vi "test_Bitfile Reload_Group Scalar to Group Static Scalar Data Type Change.vi"(8 "error in (no error)":errorcluster, 11 "TestCase in":refnum<class "FPGA Addon Bitfile Reload Unit Tests.lvclass">) -> (0 "error out":errorcluster, 3 "TestCase out":refnum<class "FPGA Addon Bitfile Reload Unit Tests.lvclass">)   [LabVIEW 2020, in "FPGA Addon Bitfile Reload Unit Tests.lvclass"]
uses:
  FPGA Addon Bitfile Reload Unit Tests.lvclass
  APIs/Scripting API/TypeDefs/Output Scalar Data.ctl
  Addon/Addon Shared/Types/FPGA Addon Data Type.ctl
  Addon/Addon Shared/SubVIs/Constants.vi
  APIs/Scripting API/Public/Bitfile Resources/Import Bitfile Scalars (Instances)/Import Scalars - all.vi
  <vilib>/addons/_JKI Toolkits/VI Tester/TestCase.llb/TestCase.lvclass
  FPGA Addon Test Class/FPGA Addon Test Class.lvclass
  APIs/Scripting API/Scripting API.lvlib
  Addon/Addon System Explorer/FPGA Addon System Explorer.lvlib
  Addon/Addon Shared/FPGA Addon Shared.lvlib
  C:/Program Files (x86)/National Instruments/LabVIEW 2020/vi.lib/addons/_JKI Toolkits/VI Tester/TestCase.llb/TestCase.lvclass
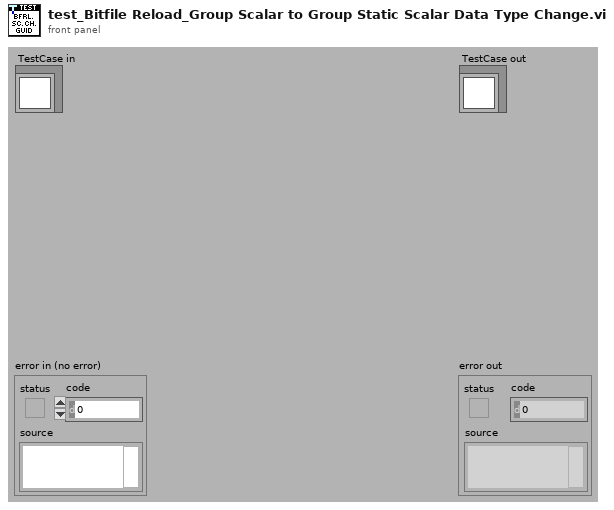
[diagram p1: front panel]
types:
  T1 = typedef "Scripting API.lvlib/Output Scalar Data.ctl" = cluster{"Bitfile Name":string, "SysDef Channel Name":string, "Imported":bool, "Data Type":T2}
  T2 = typedef "FPGA Addon Shared.lvlib/FPGA Addon Data Type.ctl" = enum8{"<Null>", "I8", "I16", "I32", "I64", "U8", "U16", "U32", "U64", "SGL", "Boolean", "Analog PWM In Settings", "Analog PWM In", "Digital PWM In Settings", "Digital PWM In", "Digital PWM Out", "Sine Out", "FXP", "FXP+/-24.5", "FXP+/-16.5", "FXP+/-32.8", "FXP+/-64.32", "FXP+/-16.7", "FXP+/-20.5", "FXP+/-27.5", "FXP+/-32.16", "FXP+16.3", "FXP+18.3", "Digital Static In", "Digital Static Out", "Digital Static In Settings", "Digital WSS Out", "Quad Encoder Settings", "Quad Encoder In", "Group"}
  T3 = typedef "Custom Device API.lvlib/Custom Device Item Ref.ctl" = u64
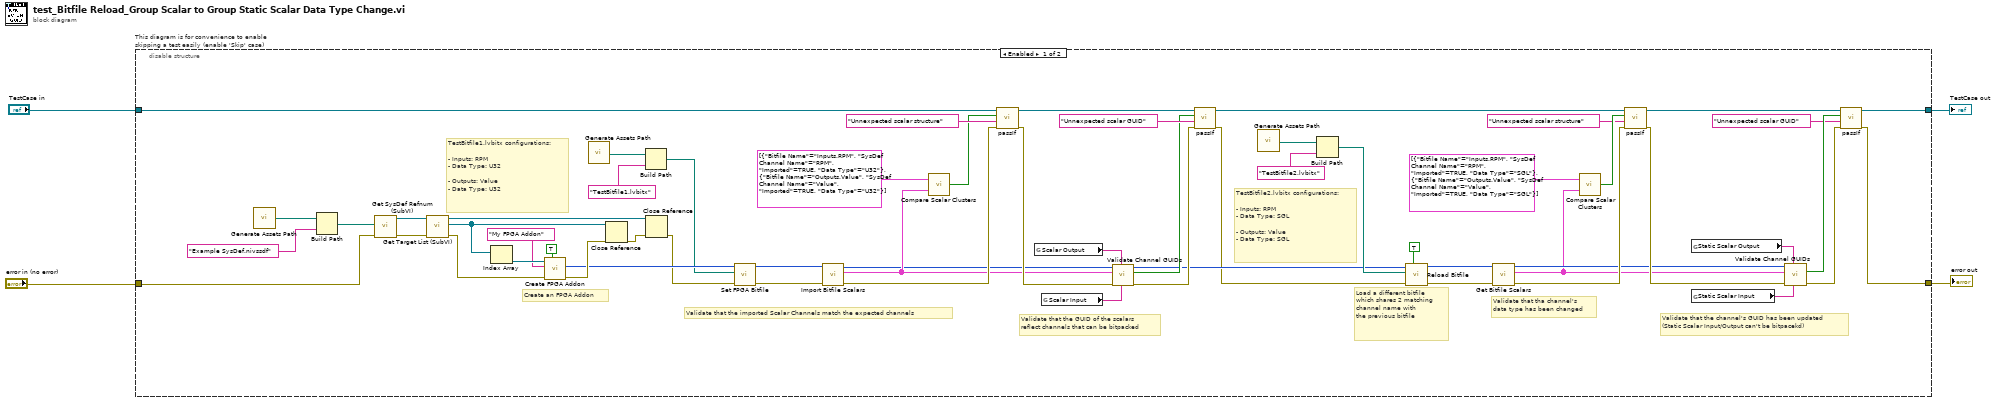
[diagram p0: block diagram]
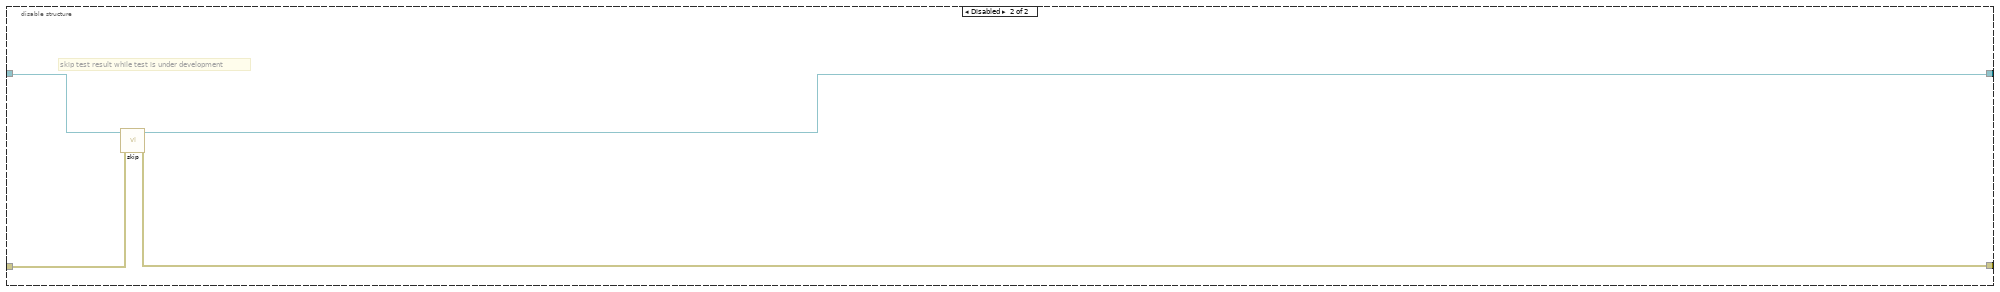
[diagram p2: hidden frame]
diagram:
  n1 = disable-structure "This diagram is for convenience to enable skipping a test easily (enable 'Skip' case)" shown="Enabled" {
    disable-tunnel: "TestCase in" -> [w32 w67]
    disable-tunnel: [w6 w65] -> w1
    disable-tunnel: [w7 w66] -> w3
    disable-tunnel: "error in (no error)" -> [w31 w64]
    frame Enabled {
      # "Validate that the GUID of the scalars\nreflect channels that can be bitpacked"
      # "Validate that the channel's GUID has been updated\n(Static Scalar Input/Output can't be bitpacekd)"
      # "TestBitfile2.lvbitx configurations:\n\n- Inputs: RPM\n- Data Type: SGL\n\n- Outputs: Value\n- Data Type: SGL"
      # "TestBitfile1.lvbitx configurations:\n\n- Inputs: RPM\n- Data Type: U32\n\n- Outputs: Value\n- Data Type: U32"
      # "Validate that tha channel's \ndata type has been changed"
      # "Load a different bitfile\nwhich shares 2 matching\nchannel name with \nthe previous bitfile"
      # "Validate that the imported Scalar Channels match the expected channels"
      # "Create an FPGA Addon"
      n2 = call "Generate Assets Path.vi"() -> ("Assets path"=w43:path)
      n3 = Build Path(base path=w43, name or relative path="Example SysDef.nivssdf") -> (appended path=w62:path)
      n4 = call "Get SysDef Refnum (SubVI).vi"("error in (no error)"=w31, "System Definition path"=w62) -> ("error out"=w58:errorcluster, "SysDef Refnum out"=w61:refnum<k24>)  [unwired: 8 in]
      n5 = call "Get Target List (SubVI).vi"("error in (no error)"=w58, "SysDef Refnum in"=w61) -> ("error out"=w57:errorcluster, "Target List Refnums"=w56:refnum<k24>[], "SysDef Refnum out"=w55:refnum<k24>)  [unwired: 7 in]
      n6 = Index Array(array=w56) -> (element=w60:refnum<k24>)  [unwired: 1 in]
      n7 = call "Create FPGA Addon.vi"("group scalars"=TRUE, "error in"=w57, "FPGA addon name"="My FPGA Addon", "target in"=w60) -> ("error out"=w53:errorcluster, "FPGA addon refnum"=w51:T3)  [unwired: 5 in, 1 out]
      n8 = call "Generate Assets Path.vi"() -> ("Assets path"=w42:path)
      n9 = Close Reference(reference=w56, error in (no error)=w53) -> (error out=w54:errorcluster)
      n10 = Build Path(base path=w42, name or relative path="TestBitfile1.lvbitx") -> (appended path=w48:path)
      n11 = Close Reference(reference=w55, error in (no error)=w54) -> (error out=w50:errorcluster)
      n12 = call "Set FPGA Bitfile.vi"("error in"=w50, "FPGA bitfile path"=w48, "FPGA addon refnum in"=w51) -> ("error out"=w47:errorcluster, "FPGA addon refnum out"=w46:T3)  [unwired: 7 in]
      n13 = call-poly "Import Bitfile Scalars.vi"("error in"=w47, "FPGA addon refnum in"=w46) -> ("error out"=w45:errorcluster, "imported bitfile scalars out"=w22:T1[], "FPGA addon refnum out"=w21:T3)  [unwired: 7 in]
      n14 = call "Compare Scalar Clusters.vi"("Target bitfile scalars in"=w22, "Reference bitfile scalars in"=T1[] [{"Bitfile Name"="Inputs.RPM", "SysDef Channel Name"="RPM", "Imported"=TRUE, "Data Type"=enum."U32"}, {"Bitfile Name"="Outputs.Value", "SysDef Channel Name"="Value", "Imported"=TRUE, "Data Type"=enum."U32"}] ("imported bitfile scalars out")) -> ("Equal ?"=w41:bool)
      n15 = call-dynamic "passIf.vi"("error in (no error)"=w45, "message (\"\")"="Unnexpected scalar structure" ("message (\"\")"), "pass"=w41, "TestCase in"=w32) -> ("error out"=w28:errorcluster, "TestCase out"=w27:refnum<class "FPGA Addon Bitfile Reload Unit Tests.lvclass">)  [unwired: 6 in]
      n16 = global read "Constants.vi" "Scalar Output"() -> (w24:string)
      n17 = global read "Constants.vi" "Scalar Input"() -> (w23:string)
      n18 = call "Validate Channel GUIDs.vi"("input GUID"=w23, "output GUID"=w24, "error in (no error)"=w28, "imported bitfile scalars in"=w22, "FPGA addon refnum in"=w21) -> ("error out"=w25:errorcluster, "valid GUIDs?"=w20:bool, "FPGA addon refnum out"=w19:T3)  [unwired: 4 in]
      n19 = call-dynamic "passIf.vi"("error in (no error)"=w25, "message (\"\")"="Unnexpected scalar GUID" ("message (\"\")"), "pass"=w20, "TestCase in"=w27) -> ("error out"=w18:errorcluster, "TestCase out"=w17:refnum<class "FPGA Addon Bitfile Reload Unit Tests.lvclass">)  [unwired: 6 in]
      n20 = call "Generate Assets Path.vi"() -> ("Assets path"=w39:path)
      n21 = Build Path(base path=w39, name or relative path="TestBitfile2.lvbitx") -> (appended path=w38:path)
      n22 = call "Reload Bitfile.vi"("Group"=TRUE, "error in (no error)"=w18, "NewVal"=w38, "Item Ref in"=w19) -> ("error out"=w37:errorcluster, "Section Ref out"=w36:T3)  [unwired: 6 in]
      n23 = call "Get Bitfile Scalars.vi"("error in"=w37, "FPGA addon refnum in"=w36) -> ("error out"=w35:errorcluster, "bitfile scalars out"=w12:T1[], "FPGA addon refnum out"=w13:T3)  [unwired: 7 in]
      n24 = call "Compare Scalar Clusters.vi"("Target bitfile scalars in"=w12, "Reference bitfile scalars in"=T1[] [{"Bitfile Name"="Inputs.RPM", "SysDef Channel Name"="RPM", "Imported"=TRUE, "Data Type"=enum."SGL"}, {"Bitfile Name"="Outputs.Value", "SysDef Channel Name"="Value", "Imported"=TRUE, "Data Type"=enum."SGL"}] ("bitfile scalars out")) -> ("Equal ?"=w34:bool)
      n25 = call-dynamic "passIf.vi"("error in (no error)"=w35, "message (\"\")"="Unnexpected scalar structure" ("message (\"\")"), "pass"=w34, "TestCase in"=w17) -> ("error out"=w14:errorcluster, "TestCase out"=w11:refnum<class "FPGA Addon Bitfile Reload Unit Tests.lvclass">)  [unwired: 6 in]
      n26 = global read "Constants.vi" "Static Scalar Output"() -> (w16:string)
      n27 = global read "Constants.vi" "Static Scalar Input"() -> (w15:string)
      n28 = call "Validate Channel GUIDs.vi"("input GUID"=w15, "output GUID"=w16, "error in (no error)"=w14, "imported bitfile scalars in"=w12, "FPGA addon refnum in"=w13) -> ("error out"=w10:errorcluster, "valid GUIDs?"=w9:bool)  [unwired: 4 in, 1 out]
      n29 = call-dynamic "passIf.vi"("error in (no error)"=w10, "message (\"\")"="Unnexpected scalar GUID" ("message (\"\")"), "pass"=w9, "TestCase in"=w11) -> ("error out"=w7:errorcluster, "TestCase out"=w6:refnum<class "FPGA Addon Bitfile Reload Unit Tests.lvclass">)  [unwired: 6 in]
    }
    frame Disabled {
      # "skip test result while test is under development"
      n30 = call <vilib>:"skip.vi"("error in (no error)"=w64, "TestCase in"=w67) -> ("error out"=w66:errorcluster, "TestCase out"=w65:refnum<class "FPGA Addon Bitfile Reload Unit Tests.lvclass">)  [unwired: 8 in]
    }
  }
  "error out" <- w3
  "TestCase out" <- w1
